vi "Calc - Splits.vi"(11 "01-02-9213":dbl[](array[numeric])) -> (2 "C.35":dbl, 3 "C.34":dbl, 5 "C.33":dbl)   [LabVIEW 2018, in "Controller (Host).lvlib"]
uses:
  Controller (Host).lvlib
  <vilib>/Analysis/baseanly.llb/Mean (DBL).vi
  <vilib>/Analysis/NI_AALBase.lvlib
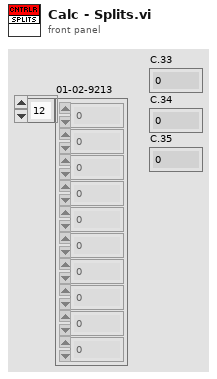
[diagram p1: front panel]
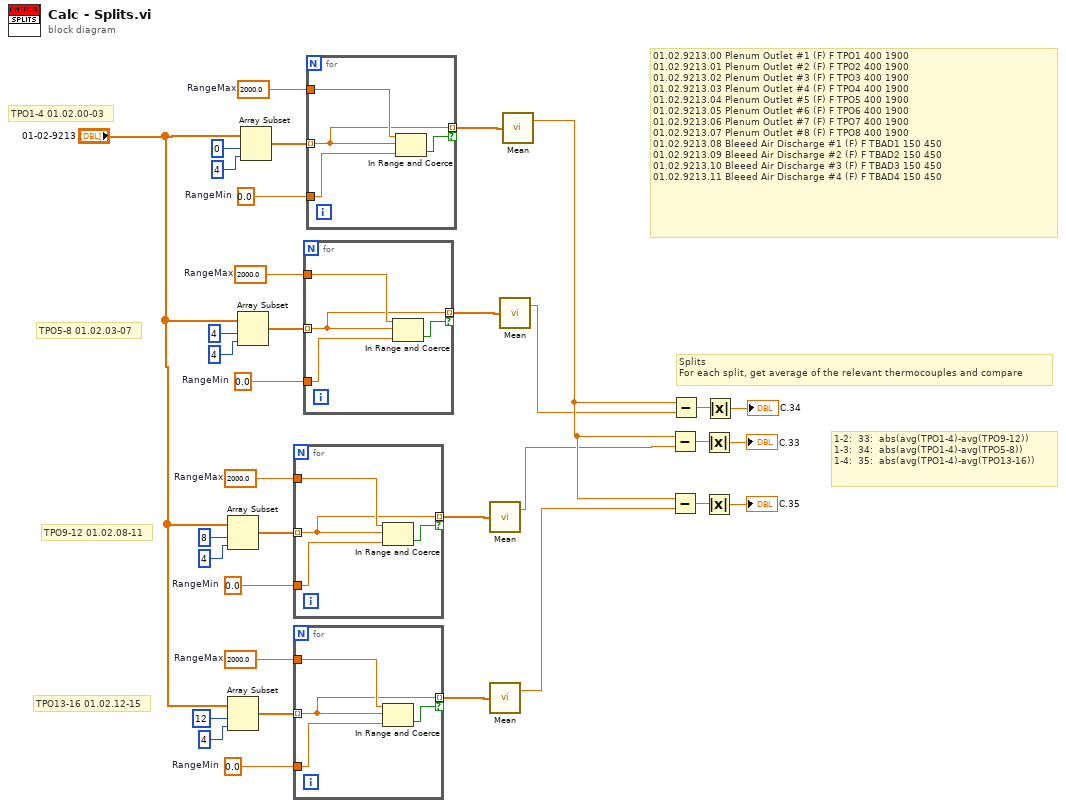
[diagram p0: block diagram]
diagram:
  w16 = 2000.0  # RangeMax
  w15 = 0.0  # RangeMin
  w19 = 2000.0  # RangeMax
  w20 = 0.0  # RangeMin
  w28 = 2000.0  # RangeMax
  w27 = 0.0  # RangeMin
  w31 = 2000.0  # RangeMax
  w32 = 0.0  # RangeMin
  # "Splits\nFor each split, get average of the relevant thermocouples and compare"
  # "01.02.9213.00\tPlenum Outlet #1 (F)\tF\tTPO1\t400\t1900\n01.02.9213.01\tPlenum Outlet #2 (F)\tF\tTPO2\t400\t1900\n01.02.9213.02\tPlenum Outlet #3 (F)\tF\tTPO3\t400\t1900\n01.02.9213.03\tPlenum Outlet #4 (F)\tF\tTPO4\t400\t1900\n01.02.9213.04\tPlenum Outlet #5 (F)\tF\tTPO5\t400\t1900\n01.02.9213.05\tPlenum Outlet #6 (F)\tF\tTPO6\t400\t1900\n01.02.9213.06\tPlenum Outlet #7 (F)\tF\tTPO7\t400\t1900\n01.02.9213.07\tPlenum Outlet #8 (F)\tF\tTPO8\t400\t1900\n01.02.9213.08\tBleeed Air Discharge #1 (F)\tF\tTBAD1\t150\t450\n01.02.9213.09\tBleeed Air Discharge #2 (F)\tF\tTBAD2\t150\t450\n01.02.9213.10\tBleeed Air Discharge #3 (F)\tF\tTBAD3\t150\t450\n01.02.9213.11\tBleeed Air Discharge #4 (F)\tF\tTBAD4\t150\t450"
  # "1-2:  33:  abs(avg(TPO1-4)-avg(TPO9-12))\n1-3:  34:  abs(avg(TPO1-4)-avg(TPO5-8))\n1-4:  35:  abs(avg(TPO1-4)-avg(TPO13-16))"
  # "TPO13-16 01.02.12-15"
  # "TPO9-12 01.02.08-11"
  # "TPO5-8 01.02.03-07"
  # "TPO1-4 01.02.00-03"
  n1 = Array Subset(array="01-02-9213", index=8, length=4) -> (w21:dbl[])
  n2 = Array Subset(array="01-02-9213", index=12, length=4) -> (w14:dbl[])
  n3 = Array Subset(array="01-02-9213", index=4, length=4) -> (w26:dbl[])
  n4 = Array Subset(array="01-02-9213", index=0, length=4) -> (w33:dbl[])
  n5 = for {
    tunnel: w21 -> [w37] mode=indexing
    tunnel: w20 -> [w38]
    tunnel: w19 -> [w39]
    tunnel: [w37] -> w18 mode=indexing if=w36
    n6 = In Range and Coerce(upper limit=w39, x=w37, lower limit=w38) -> (In Range?=w36:bool)  [unwired: 1 out]
  }
  n7 = for {
    tunnel: w14 -> [w41] mode=indexing
    tunnel: w15 -> [w42]
    tunnel: w16 -> [w43]
    tunnel: [w41] -> w17 mode=indexing if=w40
    n8 = In Range and Coerce(upper limit=w43, x=w41, lower limit=w42) -> (In Range?=w40:bool)  [unwired: 1 out]
  }
  n9 = for {
    tunnel: w26 -> [w45] mode=indexing
    tunnel: w27 -> [w46]
    tunnel: w28 -> [w47]
    tunnel: [w45] -> w29 mode=indexing if=w44
    n10 = In Range and Coerce(upper limit=w47, x=w45, lower limit=w46) -> (In Range?=w44:bool)  [unwired: 1 out]
  }
  n11 = for {
    tunnel: w33 -> [w49] mode=indexing
    tunnel: w32 -> [w50]
    tunnel: w31 -> [w51]
    tunnel: [w49] -> w30 mode=indexing if=w48
    n12 = In Range and Coerce(upper limit=w51, x=w49, lower limit=w50) -> (In Range?=w48:bool)  [unwired: 1 out]
  }
  n13 = call-poly <vilib>:"Mean.vi"("X"=w18) -> ("mean"=w1:dbl)  [unwired: 1 out]
  n14 = call-poly <vilib>:"Mean.vi"("X"=w17) -> ("mean"=w3:dbl)  [unwired: 1 out]
  n15 = call-poly <vilib>:"Mean.vi"("X"=w29) -> ("mean"=w2:dbl)  [unwired: 1 out]
  n16 = call-poly <vilib>:"Mean.vi"("X"=w30) -> ("mean"=w5:dbl)  [unwired: 1 out]
  n17 = Subtract(x=w5, y=w1) -> (x-y=w10:dbl)
  n18 = Subtract(x=w5, y=w3) -> (x-y=w6:dbl)
  n19 = Subtract(x=w5, y=w2) -> (x-y=w8:dbl)
  n20 = Absolute Value(x=w10) -> (abs(x)=→"C.33":dbl)
  n21 = Absolute Value(x=w6) -> (abs(x)=→"C.35":dbl)
  n22 = Absolute Value(x=w8) -> (abs(x)=→"C.34":dbl)
